vi "MMAxesOverlay.vi"(4 "Color Minor":u32(colorbox)=16711680, 6 "Color Major":u32(colorbox)=1351424, 8 "error in (no error)":errorcluster, 10 "cross lines":T1, 11 "Image in":T2) -> (0 "error out":errorcluster, 3 "Image out":T2)   [LabVIEW 2015]
uses:
  <vilib>/vision/Image Controls.llb/IMAQ Image.ctl
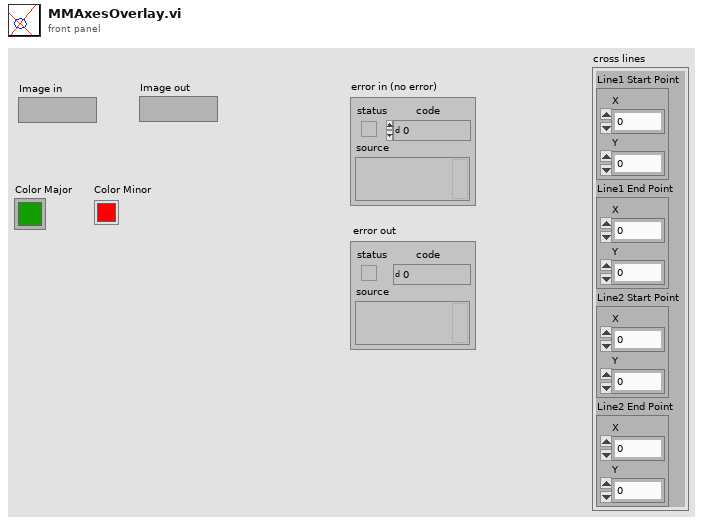
[diagram p1: front panel]
types:
  T1 = cluster{"Line1 Start Point":cluster{"X":i32, "Y":i32}, "Line1 End Point":cluster{"X":i32, "Y":i32}, "Line2 Start Point":cluster{"X":i32, "Y":i32}, "Line2 End Point":cluster{"X":i32, "Y":i32}}
  T2 = typedef "IMAQ Image.ctl" = refnum<image>
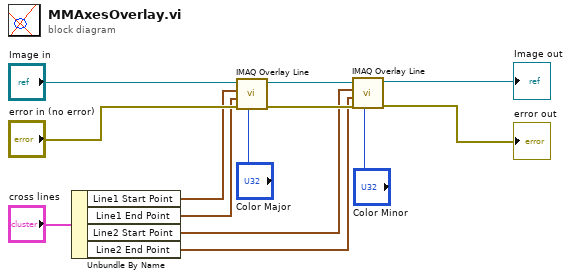
[diagram p0: block diagram]
diagram:
  n1 = Unbundle By Name("cross lines") -> ("Line1 Start Point"=w6:cluster{"X":i32, "Y":i32}, "Line1 End Point"=w5:cluster{"X":i32, "Y":i32}, "Line2 Start Point"=w4:cluster{"X":i32, "Y":i32}, "Line2 End Point"=w3:cluster{"X":i32, "Y":i32})
  n2 = call "IMAQ Overlay Line"("Color"="Color Major", "error in (no error)"="error in (no error)", "End Point"=w5, "Start Point"=w6, "Image"="Image in") -> ("error out"=w10:errorcluster, "Image Out"=w12:T2)  [unwired: 5 in]
  n3 = call "IMAQ Overlay Line"("Color"="Color Minor", "error in (no error)"=w10, "End Point"=w3, "Start Point"=w4, "Image"=w12) -> ("error out"=→"error out":errorcluster, "Image Out"=→"Image out":T2)  [unwired: 5 in]
